vi "一般动态调用.vi"(8 "error in (no error)":errorcluster, 10 "name or relative path":string="波形生成.vi") -> (0 "error out":errorcluster)   [LabVIEW 2011]
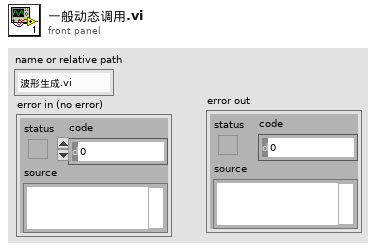
[diagram p1: front panel]
types:
  T1 = enum32{"Invalid", "Standard", "Closed", "Hidden", "Minimized", "Maximized"}
  T2 = enum32{"Bad", "Idle", "Run top level", "Running"}
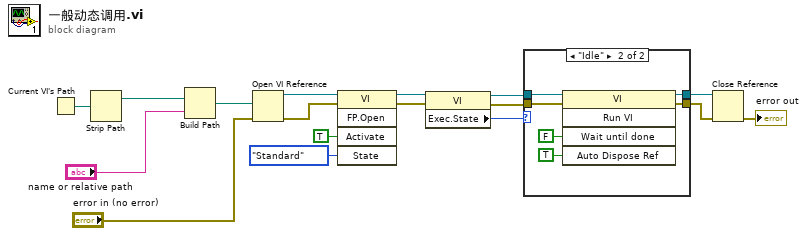
[diagram p0: block diagram]
diagram:
  n1 = Current VI's Path() -> (path=w17:path)
  n2 = Strip Path(path=w17) -> (stripped path=w16:path)  [unwired: 1 out]
  n3 = Build Path(base path=w16, name or relative path="name or relative path") -> (appended path=w14:path)
  n4 = Open VI Reference(vi path=w14, error in (no error)="error in (no error)") -> (vi reference=w13:refnum<vi>, error out=w12:errorcluster)  [unwired: 4 in]
  n5 = invoke class="VI" method="FP.Open"(reference=w13, error in=w12, "Activate"=TRUE ("Activate?"), "State"=T1."Standard") -> (reference out=w5:refnum<vi>, error out=w4:errorcluster)  [unwired: 1 in, 3 out]
  n6 = property class="VI"(reference=w5, error in=w4) -> (reference out=w2:refnum<vi>, error out=w1:errorcluster, "Exec.State"=w3:T2)
  n7 = case shown="\"Idle\"" w3 {
    tunnel: w2 -> [w19 w25]
    tunnel: w1 -> [w18 w24]
    tunnel: [w19 w21] -> w9
    tunnel: [w18 w20] -> w8
    frame "Bad", Default {
    }
    frame "Idle" {
      n8 = invoke class="VI" method="Run VI"(reference=w25, error in=w24, "Wait until done"=FALSE ("Wait Until Done"), "Auto Dispose Ref"=TRUE ("Auto Dispose Reference")) -> (reference out=w21:refnum<vi>, error out=w20:errorcluster)  [unwired: 1 in, 3 out]
    }
  }
  n9 = Close Reference(reference=w9, error in (no error)=w8) -> (error out=→"error out":errorcluster)
